vi "test lijndetectie.vi"() -> ()   [LabVIEW 2019]
uses:
  <vilib>/myRIO/Instrument Drivers/Onboard IO/AI/typedefs/AI Reference.ctl
  <vilib>/myRIO/Common/Instrument Driver Framework/Utilities/typedefs/myRIO Generic Hardware Reference.ctl
  <vilib>/myRIO/Common/Instrument Driver Framework/Utilities/typedefs/Hardware Version Enum.ctl
  <vilib>/myRIO/Common/Instrument Driver Framework/Utilities/typedefs/myRIO v1.0 Reference.ctl
  <vilib>/myRIO/Common/Instrument Driver Framework/Utilities/typedefs/Generic FPGA Reference.ctl
  <vilib>/myRIO/Common/Instrument Driver Framework/myRIO v1.0/AI/typedefs/AI Channels List.ctl
  <vilib>/myRIO/Common/Instrument Driver Framework/myRIO v1.0/AI/typedefs/AI Channels Enum.ctl
  <vilib>/myRIO/Common/Instrument Driver Framework/Utilities/typedefs/Analog Scaling Constants List.ctl
  <vilib>/myRIO/Common/Instrument Driver Framework/Utilities/typedefs/Analog Scaling Constants.ctl
  <vilib>/userDefined/High Color/nirio_resource_hc.ctl
  <vilib>/myRIO/Common/Instrument Driver Framework/Utilities/vis/Is FPGA Ref Available.vi
  <vilib>/myRIO/Common/Instrument Driver Framework/myRIO v1.0/AI/vis/myRIO v1.1 Open AI.vi
  <vilib>/myRIO/Instrument Drivers/Onboard IO/AI/vis/Read.vi
  <vilib>/myRIO/Common/Instrument Driver Framework/Utilities/vis/Validate Channels.vi
  <vilib>/myRIO/Common/Instrument Driver Framework/myRIO v1.0/AI/vis/myRIO v1.0 Reserve AI.vi
  <vilib>/myRIO/Common/Instrument Driver Framework/myRIO v1.0/AI/vis/myRIO v1.0 Build MUX Configuration AI.vi
  <vilib>/myRIO/Common/Instrument Driver Framework/myRIO v1.0/Resource Manager/vis/myRIO v1.0 Reserve Channel List.vi
  <vilib>/myRIO/Common/Instrument Driver Framework/myRIO v1.0/Resource Manager/vis/myRIO v1.0 Reserve Channel.vi
  <vilib>/myRIO/Common/Instrument Driver Framework/myRIO v1.0/Resource Manager/vis/myRIO v1.0 Unreserve Channel.vi
  <vilib>/myRIO/Common/Instrument Driver Framework/myRIO v1.0/Resource Manager/vis/myRIO v1.0 Build Mutex Name.vi
  <vilib>/Utility/VariantDataType/GetNumericInfo.vi
  <vilib>/Utility/error.llb/Error Cluster From Error Code.vi
  <vilib>/myRIO/Common/Instrument Driver Framework/myRIO v1.0/myRIO v1.1 Open.vi
  <vilib>/myRIO/Common/Instrument Driver Framework/myRIO v1.0/AI/vis/myRIO v1.0 Get Scaling Constants AI.vi
  <vilib>/myRIO/Common/Instrument Driver Framework/Utilities/vis/IO Manager.vi
  <vilib>/myRIO/Common/Instrument Driver Framework/Utilities/vis/Configuration Manager.vi
  <vilib>/myRIO/Common/Instrument Driver Framework/myRIO v1.0/myRIO v1.0 Close.vi
  <vilib>/myRIO/Common/Instrument Driver Framework/myRIO v1.0/AI/vis/myRIO v1.0 Read AI.vi
  <vilib>/myRIO/Express VI/Onboard IO/AI/AI Express VI.xnode
  <vilib>/myRIO/Instrument Drivers/Onboard IO/AI/vis/myRIO AI Open.xnode
  <vilib>/myRIO/Instrument Drivers/Onboard IO/AI/AI.lvlib
panel:
  out "analoog":dbl[](array[numeric])
  out "motor  stilleggen":bool
  out "motor zwak links sneller":bool
  out "motor naar rechts sneller":bool
  out "motor zeer sterk rechts sneller":bool
  out "motoren sterk links sneller":bool
  out "motor sterk rechts sneller":bool
  out "motor zwak naar rechts sneller":bool
  out "motor  zeer sterk links sneller":bool
  out "motor naar links sneller":bool
  out "digitaal":i32[](array[numeric])
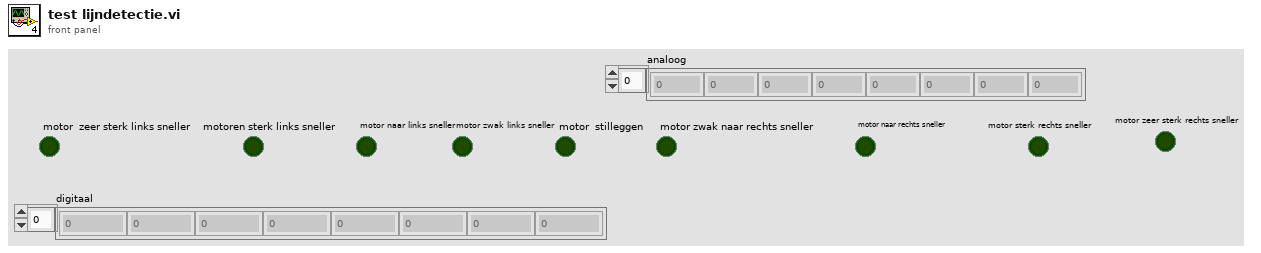
[diagram p1: front panel]
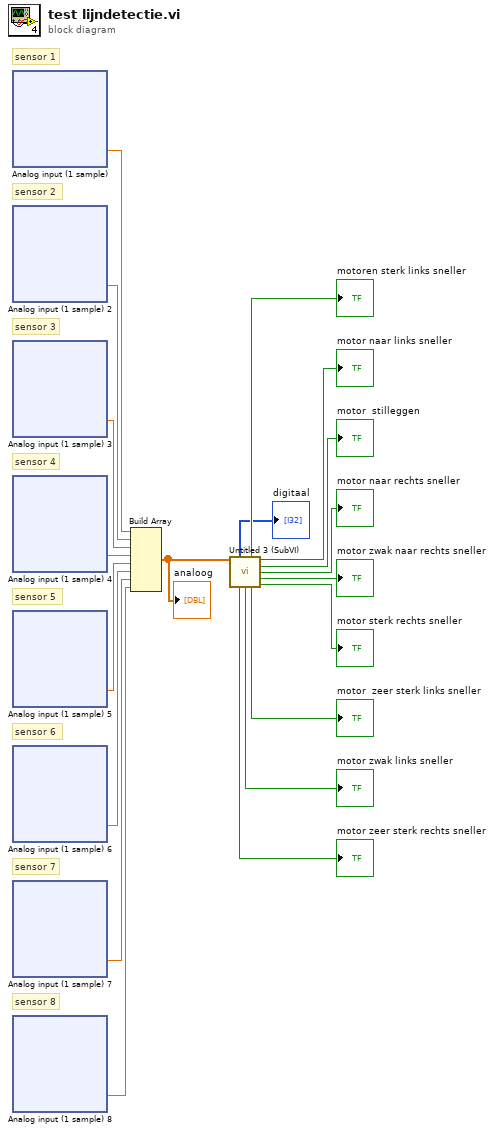
[diagram p0: block diagram]
diagram:
  # "sensor 8"
  # "sensor 7"
  # "sensor 6"
  # "sensor 5"
  # "sensor 4"
  # "sensor 3"
  # "sensor 2"
  # "sensor 1"
  n1 = xnode "Analog input (1 sample)"() -> ("A/AI3 (Pin 9)"=w8:dbl)  [unwired: 1 in, 1 out]
  n2 = xnode "Analog input (1 sample) 2"() -> ("A/AI2 (Pin 7)"=w7:dbl)  [unwired: 1 in, 1 out]
  n3 = xnode "Analog input (1 sample) 3"() -> ("A/AI1 (Pin 5)"=w6:dbl)  [unwired: 1 in, 1 out]
  n4 = xnode "Analog input (1 sample) 4"() -> ("A/AI0 (Pin 3)"=w5:dbl)  [unwired: 1 in, 1 out]
  n5 = xnode "Analog input (1 sample) 5"() -> ("B/AI3 (Pin 9)"=w4:dbl)  [unwired: 1 in, 1 out]
  n6 = xnode "Analog input (1 sample) 6"() -> ("B/AI2 (Pin 7)"=w3:dbl)  [unwired: 1 in, 1 out]
  n7 = xnode "Analog input (1 sample) 7"() -> ("A/AI1 (Pin 5)"=w2:dbl)  [unwired: 1 in, 1 out]
  n8 = xnode "Analog input (1 sample) 8"() -> ("B/AI0 (Pin 3)"=w1:dbl)  [unwired: 1 in, 1 out]
  n9 = Build Array(w8, w7, w6, w5, w4, w3, w2, w1) -> (w9:dbl[])
  "analoog" <- w9
  n10 = call "Untitled 3 (SubVI).vi"("input array   in"=w9) -> ("Array"=→"digitaal":i32[], "motoren sterk links sneller"=→"motoren sterk links sneller":bool, "motor naar links sneller"=→"motor naar links sneller":bool, "motor  stilleggen"=→"motor  stilleggen":bool, "motor naar rechts sneller"=→"motor naar rechts sneller":bool, "motor zwak naar rechts sneller"=→"motor zwak naar rechts sneller":bool, "motor zeer sterk rechts sneller"=→"motor zeer sterk rechts sneller":bool, "motor zwak links sneller"=→"motor zwak links sneller":bool, "motor  zeer sterk links sneller"=→"motor  zeer sterk links sneller":bool, "motor sterk rechts sneller"=→"motor sterk rechts sneller":bool)  [unwired: 5 in]
